vi "Front_Panel_Basic.vi"() -> ()   [LabVIEW 2015]
uses:
  Program Files (x86)/National Instruments/LabVIEW 2012/examples/Vision/2. Functions/Caliper/Control 1.ctl
panel:
  in  "Reset Sensor":bool
  in  "Set all":bool
  in  "Digital Offset Get":bool caption="Line Period Get"
  in  "Digital Offset Set":bool caption="Line Period Set"
  in  "Digital Offset":i16 min=-4096 max=4095 step=1
  in  "Digital Gain Get":bool caption="Line Period Get"
  in  "Digital Gain Set":bool caption="Line Period Set"
  in  "Digital Gain":i16 min=0 max=1791 step=1
  in  "Analog Gain Get":bool caption="Line Period Get"
  in  "Analog Gain Set":bool caption="Line Period Set"
  in  "Analog Gain":u16 max=2
  in  "Trigger Modes Get":bool caption="Line Period Get"
  in  "Trigger Modes Set":bool caption="Line Period Set"
  in  "Trigger Modes":u16 max=3
  in  "Exposure Time Get":bool caption="Line Period Get"
  in  "Exposure Time Set":bool caption="Line Period Set"
  in  "Exposure Time":u16 min=1
  in  "Line Period Get":bool
  in  "Line Period Set":bool
  in  "Line Period":T1=1 min=1 step=1
  out "Sensor width":string
  out "Firmware version":string
  out "User defined name":string
  out "Serial number":string
  out "Manufactuer info":string
  out "Device version":string
  out "Model Name":string
  out "Manufacturer name":string
  in  "Download Button":bool
  in  "EXIT":bool
  in  "Get All":bool
  out "IMAQ Session Out":refnum<k11>
  out "Error Output":errorcluster
  in  "error in (no error)":errorcluster
  # "Line period from 1 (0.01us) to 65535 (655,35 us) with\nstep size 1 (0.01us)."
  # "0: x1.0 gain\n1: x2.0 gain\n2: x4.0 gain"
  # "Exposure time from 1 (0.01us) to 65535 (655,35 us) with step size 1 (0.01us)."
  # "Digial gain from x1.0 (0) to x7.9961 (1791), with a \nstep size of 0x0.0039 (1)"
  # "0: Internal line trigger with programmable exposure time and line period\n1: Internal line trigger with max exporure time and programmable line period\n2: External line trigger with programmable exposure time\n3: External line trigger with maximum exposure time"
  # "Digial offset from -4096 to 4095 with a step size of 1\nin 12-bit mode.\nIn 11-bit mode, offset will be divided by 2.\nIn 10-bit mode, offset will be divided by 4."
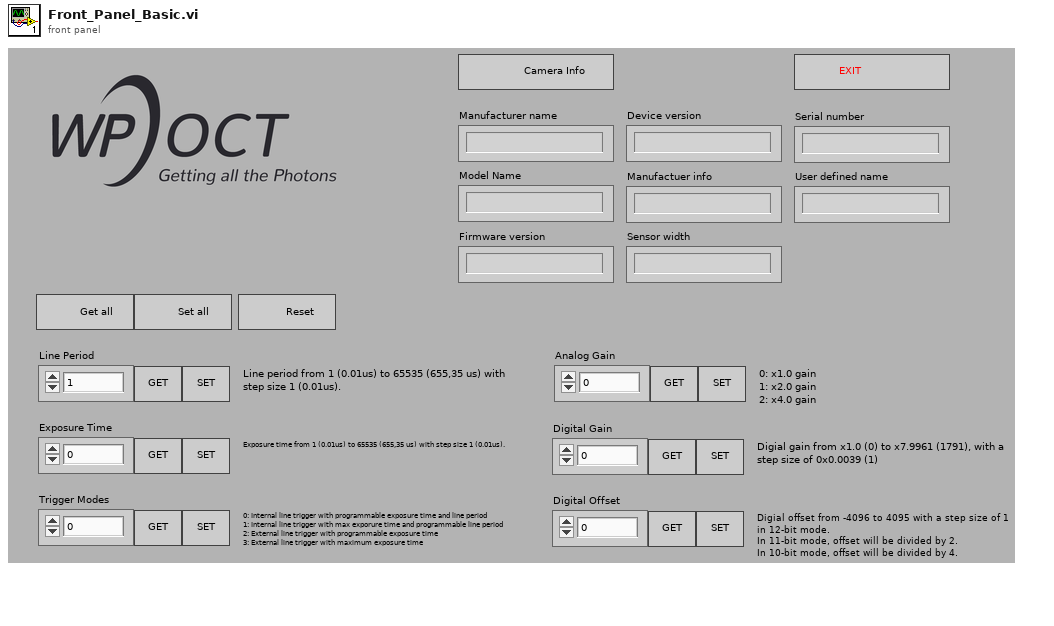
[diagram p1: front panel]
types:
  T1 = typedef "Control 1.ctl" = u16
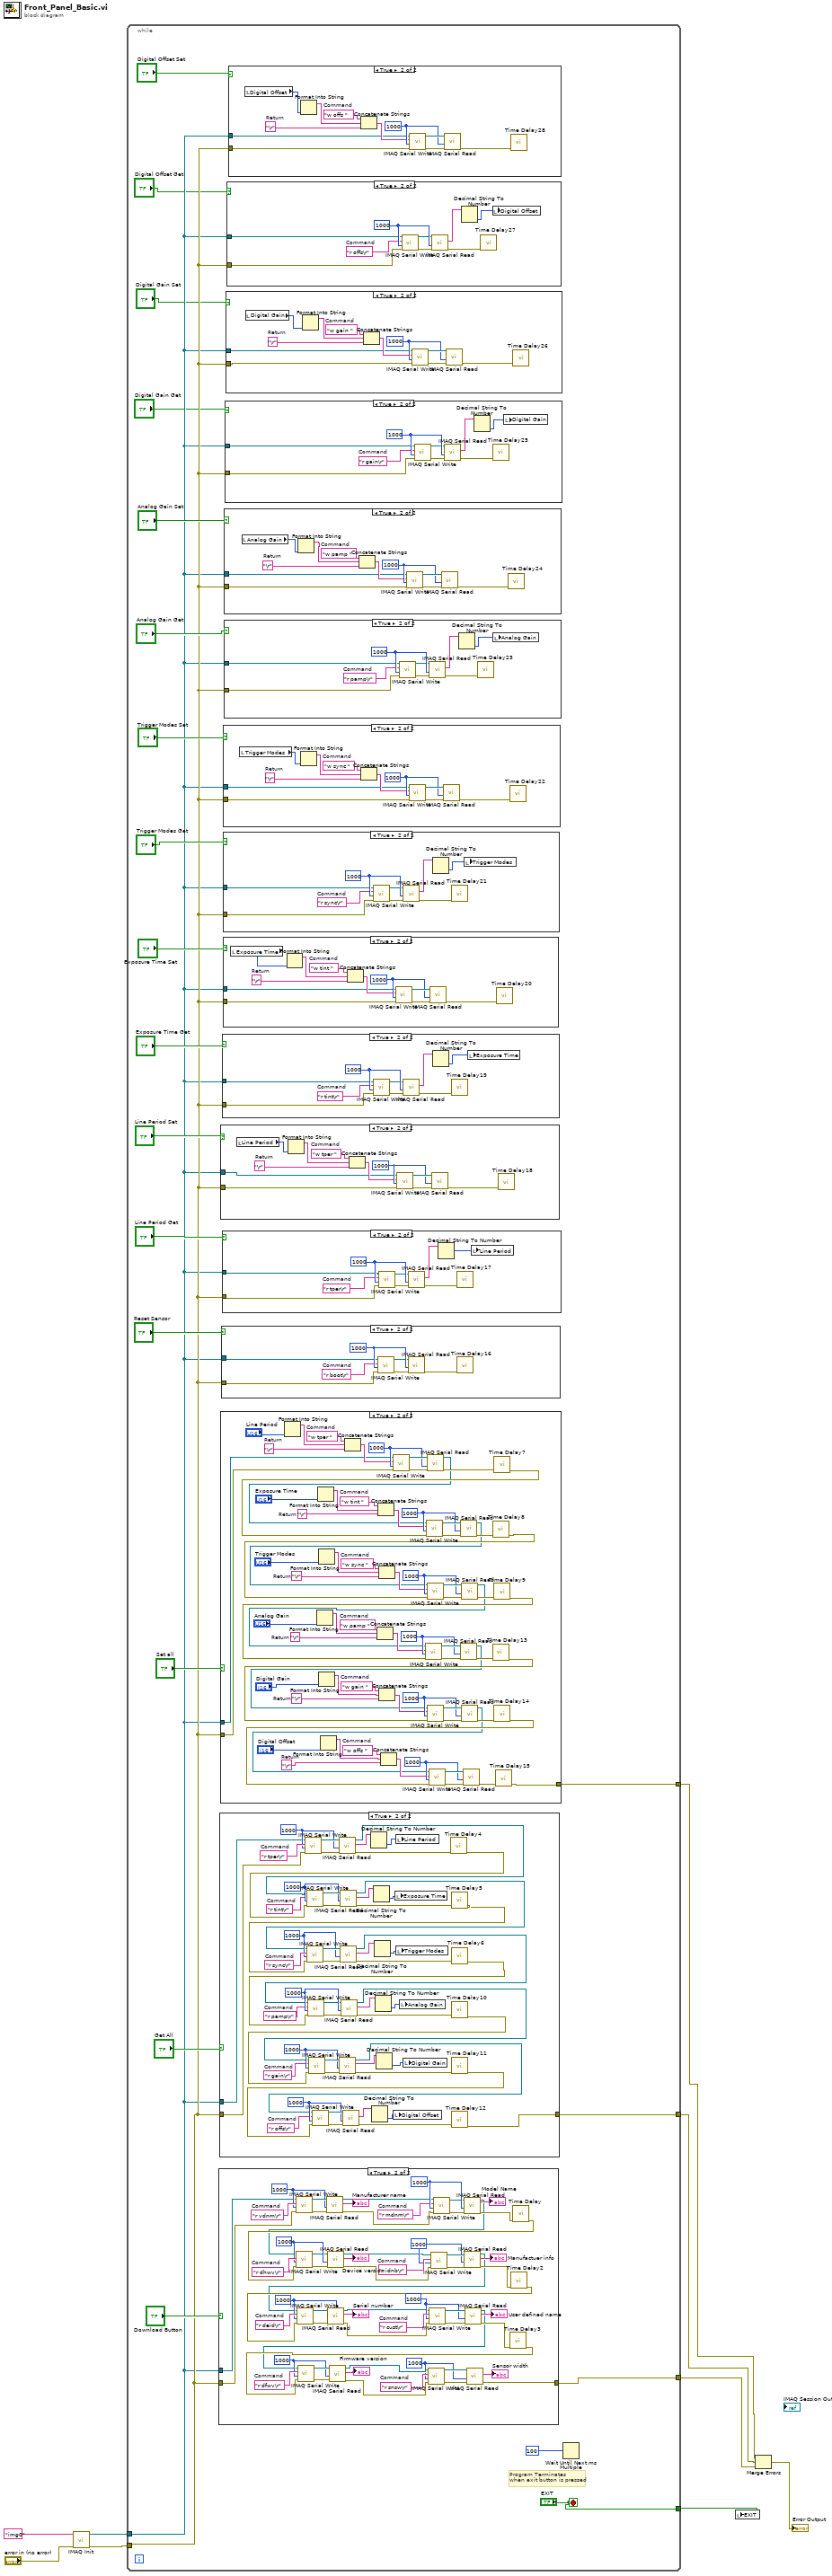
[diagram p0: block diagram]
diagram:
  n1 = call <vilib>:"IMAQ Init.vi"("error in (no error)"="error in (no error)", "Interface Name"="img0") -> ("error out"=w7:errorcluster, "IMAQ Session Out"=w8:refnum<k11>)  [unwired: 8 in]
  n2 = while {
    tunnel: w8 -> [w14]
    tunnel: w7 -> [w15]
    tunnel: ["EXIT"] -> w4
    tunnel: [w29] -> w3
    tunnel: [w26] -> w2
    tunnel: [w25] -> w1
    stop <- "EXIT" stop-if-true
    # "Program Terminates\nwhen exit button is pressed"
    n3 = case shown="True" "Download Button" {
      tunnel: w15 -> [w284 w307]
      tunnel: [w284 w285] -> w29
      tunnel: w14 -> [_ w306]
      frame False {
      }
      frame True {
        w310 = "r vdnm\r"  # Command
        w308 = 1000
        w316 = 1000
        w315 = "r mdnm\r"  # Command
        w320 = "r dhwv\r"  # Command
        w319 = 1000
        w322 = "r idnb\r"  # Command
        w321 = 1000
        w326 = 1000
        w327 = "r deid\r"  # Command
        w334 = "r cust\r"  # Command
        w331 = 1000
        w340 = "r dfwv\r"  # Command
        w336 = 1000
        w343 = "r snsw\r"  # Command
        w286 = 1000
        n4 = call <vilib>:"IMAQ Serial Write.vi"("error in (no error)"=w307, "Timeout"=w308, "String to write"=w310, "IMAQ Session In"=w306) -> ("error out"=w309:errorcluster, "IMAQ Session Out"=w311:refnum<k11>)  [unwired: 4 in]
        n5 = call <vilib>:"IMAQ Serial Read.vi"("error in (no error)"=w309, "Timeout"=w308, "IMAQ Session In"=w311) -> ("error out"=w303:errorcluster, "String Read"=→"Manufacturer name":string, "IMAQ Session Out"=w304:refnum<k11>)  [unwired: 3 in, 1 out]
        n6 = call <vilib>:"IMAQ Serial Write.vi"("error in (no error)"=w303, "Timeout"=w316, "String to write"=w315, "IMAQ Session In"=w304) -> ("error out"=w313:errorcluster, "IMAQ Session Out"=w312:refnum<k11>)  [unwired: 4 in]
        n7 = call <vilib>:"IMAQ Serial Read.vi"("error in (no error)"=w313, "Timeout"=w316, "IMAQ Session In"=w312) -> ("error out"=w302:errorcluster, "String Read"=→"Model Name":string, "IMAQ Session Out"=w300:refnum<k11>)  [unwired: 3 in, 1 out]
        n8 = call "Time Delay"("error in (no error)"=w302) -> ("error out"=w301:errorcluster)  [unwired: 10 in]
        n9 = call <vilib>:"IMAQ Serial Write.vi"("error in (no error)"=w301, "Timeout"=w319, "String to write"=w320, "IMAQ Session In"=w300) -> ("error out"=w318:errorcluster, "IMAQ Session Out"=w317:refnum<k11>)  [unwired: 4 in]
        n10 = call <vilib>:"IMAQ Serial Read.vi"("error in (no error)"=w318, "Timeout"=w319, "IMAQ Session In"=w317) -> ("error out"=w298:errorcluster, "String Read"=→"Device version":string, "IMAQ Session Out"=w297:refnum<k11>)  [unwired: 3 in, 1 out]
        n11 = call <vilib>:"IMAQ Serial Write.vi"("error in (no error)"=w298, "Timeout"=w321, "String to write"=w322, "IMAQ Session In"=w297) -> ("error out"=w323:errorcluster, "IMAQ Session Out"=w325:refnum<k11>)  [unwired: 4 in]
        n12 = call <vilib>:"IMAQ Serial Read.vi"("error in (no error)"=w323, "Timeout"=w321, "IMAQ Session In"=w325) -> ("error out"=w296:errorcluster, "String Read"=→"Manufactuer info":string, "IMAQ Session Out"=w294:refnum<k11>)  [unwired: 3 in, 1 out]
        n13 = call "Time Delay2"("error in (no error)"=w296) -> ("error out"=w295:errorcluster)  [unwired: 10 in]
        n14 = call <vilib>:"IMAQ Serial Write.vi"("error in (no error)"=w295, "Timeout"=w326, "String to write"=w327, "IMAQ Session In"=w294) -> ("error out"=w328:errorcluster, "IMAQ Session Out"=w329:refnum<k11>)  [unwired: 4 in]
        n15 = call <vilib>:"IMAQ Serial Read.vi"("error in (no error)"=w328, "Timeout"=w326, "IMAQ Session In"=w329) -> ("error out"=w289:errorcluster, "String Read"=→"Serial number":string, "IMAQ Session Out"=w293:refnum<k11>)  [unwired: 3 in, 1 out]
        n16 = call <vilib>:"IMAQ Serial Write.vi"("error in (no error)"=w289, "Timeout"=w331, "String to write"=w334, "IMAQ Session In"=w293) -> ("error out"=w332:errorcluster, "IMAQ Session Out"=w333:refnum<k11>)  [unwired: 4 in]
        n17 = call <vilib>:"IMAQ Serial Read.vi"("error in (no error)"=w332, "Timeout"=w331, "IMAQ Session In"=w333) -> ("error out"=w292:errorcluster, "String Read"=→"User defined name":string, "IMAQ Session Out"=w290:refnum<k11>)  [unwired: 3 in, 1 out]
        n18 = call "Time Delay3"("error in (no error)"=w292) -> ("error out"=w291:errorcluster)  [unwired: 10 in]
        n19 = call <vilib>:"IMAQ Serial Write.vi"("error in (no error)"=w291, "Timeout"=w336, "String to write"=w340, "IMAQ Session In"=w290) -> ("error out"=w337:errorcluster, "IMAQ Session Out"=w338:refnum<k11>)  [unwired: 4 in]
        n20 = call <vilib>:"IMAQ Serial Read.vi"("error in (no error)"=w337, "Timeout"=w336, "IMAQ Session In"=w338) -> ("error out"=w288:errorcluster, "String Read"=→"Firmware version":string, "IMAQ Session Out"=w287:refnum<k11>)  [unwired: 3 in, 1 out]
        n21 = call <vilib>:"IMAQ Serial Write.vi"("error in (no error)"=w288, "Timeout"=w286, "String to write"=w343, "IMAQ Session In"=w287) -> ("error out"=w342:errorcluster, "IMAQ Session Out"=w341:refnum<k11>)  [unwired: 4 in]
        n22 = call <vilib>:"IMAQ Serial Read.vi"("error in (no error)"=w342, "Timeout"=w286, "IMAQ Session In"=w341) -> ("error out"=w285:errorcluster, "String Read"=→"Sensor width":string)  [unwired: 3 in, 2 out]
      }
    }
    n23 = case shown="True" "Get All" {
      tunnel: w15 -> [w228 w279]
      tunnel: [w228 w234] -> w26
      tunnel: w14 -> [_ w278]
      frame False {
      }
      frame True {
        w236 = "r offs\r"  # Command
        w237 = 1000
        w260 = "r gain\r"  # Command
        w262 = 1000
        w265 = "r pamp\r"  # Command
        w266 = 1000
        w269 = "r sync\r"  # Command
        w250 = 1000
        w272 = "r tint\r"  # Command
        w274 = 1000
        w282 = "r tper\r"  # Command
        w280 = 1000
        n24 = call <vilib>:"IMAQ Serial Write.vi"("error in (no error)"=w279, "Timeout"=w280, "String to write"=w282, "IMAQ Session In"=w278) -> ("error out"=w281:errorcluster, "IMAQ Session Out"=w283:refnum<k11>)  [unwired: 4 in]
        n25 = call <vilib>:"IMAQ Serial Read.vi"("error in (no error)"=w281, "Timeout"=w280, "IMAQ Session In"=w283) -> ("error out"=w277:errorcluster, "String Read"=w241:string, "IMAQ Session Out"=w240:refnum<k11>)  [unwired: 3 in, 1 out]
        n26 = Decimal String To Number(string=w241) -> (number=w229:i32)  [unwired: 2 in, 1 out]
        n27 = local write "Line Period"(w229) -> ()
        n28 = call "Time Delay4"("error in (no error)"=w277) -> ("error out"=w242:errorcluster)  [unwired: 10 in]
        n29 = call <vilib>:"IMAQ Serial Write.vi"("error in (no error)"=w242, "Timeout"=w274, "String to write"=w272, "IMAQ Session In"=w240) -> ("error out"=w275:errorcluster, "IMAQ Session Out"=w276:refnum<k11>)  [unwired: 4 in]
        n30 = call <vilib>:"IMAQ Serial Read.vi"("error in (no error)"=w275, "Timeout"=w274, "IMAQ Session In"=w276) -> ("error out"=w273:errorcluster, "String Read"=w245:string, "IMAQ Session Out"=w243:refnum<k11>)  [unwired: 3 in, 1 out]
        n31 = Decimal String To Number(string=w245) -> (number=w244:i32)  [unwired: 2 in, 1 out]
        n32 = local write "Exposure Time"(w244) -> ()
        n33 = call "Time Delay5"("error in (no error)"=w273) -> ("error out"=w249:errorcluster)  [unwired: 10 in]
        n34 = call <vilib>:"IMAQ Serial Write.vi"("error in (no error)"=w249, "Timeout"=w250, "String to write"=w269, "IMAQ Session In"=w243) -> ("error out"=w270:errorcluster, "IMAQ Session Out"=w271:refnum<k11>)  [unwired: 4 in]
        n35 = call <vilib>:"IMAQ Serial Read.vi"("error in (no error)"=w270, "Timeout"=w250, "IMAQ Session In"=w271) -> ("error out"=w248:errorcluster, "String Read"=w247:string, "IMAQ Session Out"=w246:refnum<k11>)  [unwired: 3 in, 1 out]
        n36 = Decimal String To Number(string=w247) -> (number=w268:i32)  [unwired: 2 in, 1 out]
        n37 = local write "Trigger Modes"(w268) -> ()
        n38 = call "Time Delay6"("error in (no error)"=w248) -> ("error out"=w251:errorcluster)  [unwired: 10 in]
        n39 = call <vilib>:"IMAQ Serial Write.vi"("error in (no error)"=w251, "Timeout"=w266, "String to write"=w265, "IMAQ Session In"=w246) -> ("error out"=w267:errorcluster, "IMAQ Session Out"=w257:refnum<k11>)  [unwired: 4 in]
        n40 = call <vilib>:"IMAQ Serial Read.vi"("error in (no error)"=w267, "Timeout"=w266, "IMAQ Session In"=w257) -> ("error out"=w253:errorcluster, "String Read"=w255:string, "IMAQ Session Out"=w254:refnum<k11>)  [unwired: 3 in, 1 out]
        n41 = Decimal String To Number(string=w255) -> (number=w256:i32)  [unwired: 2 in, 1 out]
        n42 = local write "Analog Gain"(w256) -> ()
        n43 = call "Time Delay10"("error in (no error)"=w253) -> ("error out"=w252:errorcluster)  [unwired: 10 in]
        n44 = call <vilib>:"IMAQ Serial Write.vi"("error in (no error)"=w252, "Timeout"=w262, "String to write"=w260, "IMAQ Session In"=w254) -> ("error out"=w263:errorcluster, "IMAQ Session Out"=w264:refnum<k11>)  [unwired: 4 in]
        n45 = call <vilib>:"IMAQ Serial Read.vi"("error in (no error)"=w263, "Timeout"=w262, "IMAQ Session In"=w264) -> ("error out"=w261:errorcluster, "String Read"=w259:string, "IMAQ Session Out"=w232:refnum<k11>)  [unwired: 3 in, 1 out]
        n46 = Decimal String To Number(string=w259) -> (number=w258:i32)  [unwired: 2 in, 1 out]
        n47 = local write "Digital Gain"(w258) -> ()
        n48 = call "Time Delay11"("error in (no error)"=w261) -> ("error out"=w233:errorcluster)  [unwired: 10 in]
        n49 = call <vilib>:"IMAQ Serial Write.vi"("error in (no error)"=w233, "Timeout"=w237, "String to write"=w236, "IMAQ Session In"=w232) -> ("error out"=w238:errorcluster, "IMAQ Session Out"=w239:refnum<k11>)  [unwired: 4 in]
        n50 = call <vilib>:"IMAQ Serial Read.vi"("error in (no error)"=w238, "Timeout"=w237, "IMAQ Session In"=w239) -> ("error out"=w235:errorcluster, "String Read"=w231:string)  [unwired: 3 in, 2 out]
        n51 = Decimal String To Number(string=w231) -> (number=w230:i32)  [unwired: 2 in, 1 out]
        n52 = local write "Digital Offset"(w230) -> ()
        n53 = call "Time Delay12"("error in (no error)"=w235) -> ("error out"=w234:errorcluster)  [unwired: 10 in]
      }
    }
    n54 = case shown="True" "Set all" {
      tunnel: w15 -> [w160 w219]
      tunnel: [w160 w161] -> w25
      tunnel: w14 -> [_ w220]
      frame False {
      }
      frame True {
        w163 = "\r"  # Return
        w169 = "w offs "  # Command
        w170 = 1000
        w175 = "\r"  # Return
        w180 = "w gain "  # Command
        w181 = 1000
        w188 = "\r"  # Return
        w191 = "w pamp "  # Command
        w192 = 1000
        w196 = "\r"  # Return
        w201 = "w sync "  # Command
        w203 = 1000
        w213 = "\r"  # Return
        w211 = "w tint "  # Command
        w214 = 1000
        w224 = "\r"  # Return
        w222 = "w tper "  # Command
        w225 = 1000
        n55 = Format Into String("Line Period") -> (resulting string=w223:string)  [unwired: 3 in, 1 out]
        n56 = Format Into String("Analog Gain") -> (resulting string=w185:string)  [unwired: 3 in, 1 out]
        n57 = Format Into String("Exposure Time") -> (resulting string=w212:string)  [unwired: 3 in, 1 out]
        n58 = Format Into String("Trigger Modes") -> (resulting string=w202:string)  [unwired: 3 in, 1 out]
        n59 = Format Into String("Digital Gain") -> (resulting string=w174:string)  [unwired: 3 in, 1 out]
        n60 = Format Into String("Digital Offset") -> (resulting string=w162:string)  [unwired: 3 in, 1 out]
        n61 = Concatenate Strings(w222, w223, w224) -> (w221:string)
        n62 = Concatenate Strings(w191, w185, w188) -> (w190:string)
        n63 = Concatenate Strings(w211, w212, w213) -> (w210:string)
        n64 = Concatenate Strings(w201, w202, w196) -> (w200:string)
        n65 = Concatenate Strings(w180, w174, w175) -> (w179:string)
        n66 = Concatenate Strings(w169, w162, w163) -> (w168:string)
        n67 = call <vilib>:"IMAQ Serial Write.vi"("error in (no error)"=w219, "Timeout"=w225, "String to write"=w221, "IMAQ Session In"=w220) -> ("error out"=w226:errorcluster, "IMAQ Session Out"=w227:refnum<k11>)  [unwired: 4 in]
        n68 = call <vilib>:"IMAQ Serial Read.vi"("error in (no error)"=w226, "Timeout"=w225, "IMAQ Session In"=w227) -> ("error out"=w217:errorcluster, "IMAQ Session Out"=w206:refnum<k11>)  [unwired: 3 in, 2 out]
        n69 = call "Time Delay7"("error in (no error)"=w217) -> ("error out"=w207:errorcluster)  [unwired: 10 in]
        n70 = call <vilib>:"IMAQ Serial Write.vi"("error in (no error)"=w207, "Timeout"=w214, "String to write"=w210, "IMAQ Session In"=w206) -> ("error out"=w215:errorcluster, "IMAQ Session Out"=w216:refnum<k11>)  [unwired: 4 in]
        n71 = call <vilib>:"IMAQ Serial Read.vi"("error in (no error)"=w215, "Timeout"=w214, "IMAQ Session In"=w216) -> ("error out"=w209:errorcluster, "IMAQ Session Out"=w197:refnum<k11>)  [unwired: 3 in, 2 out]
        n72 = call "Time Delay8"("error in (no error)"=w209) -> ("error out"=w198:errorcluster)  [unwired: 10 in]
        n73 = call <vilib>:"IMAQ Serial Write.vi"("error in (no error)"=w198, "Timeout"=w203, "String to write"=w200, "IMAQ Session In"=w197) -> ("error out"=w204:errorcluster, "IMAQ Session Out"=w205:refnum<k11>)  [unwired: 4 in]
        n74 = call <vilib>:"IMAQ Serial Read.vi"("error in (no error)"=w204, "Timeout"=w203, "IMAQ Session In"=w205) -> ("error out"=w199:errorcluster, "IMAQ Session Out"=w186:refnum<k11>)  [unwired: 3 in, 2 out]
        n75 = call "Time Delay9"("error in (no error)"=w199) -> ("error out"=w187:errorcluster)  [unwired: 10 in]
        n76 = call <vilib>:"IMAQ Serial Write.vi"("error in (no error)"=w187, "Timeout"=w192, "String to write"=w190, "IMAQ Session In"=w186) -> ("error out"=w193:errorcluster, "IMAQ Session Out"=w194:refnum<k11>)  [unwired: 4 in]
        n77 = call <vilib>:"IMAQ Serial Read.vi"("error in (no error)"=w193, "Timeout"=w192, "IMAQ Session In"=w194) -> ("error out"=w189:errorcluster, "IMAQ Session Out"=w176:refnum<k11>)  [unwired: 3 in, 2 out]
        n78 = call "Time Delay13"("error in (no error)"=w189) -> ("error out"=w177:errorcluster)  [unwired: 10 in]
        n79 = call <vilib>:"IMAQ Serial Write.vi"("error in (no error)"=w177, "Timeout"=w181, "String to write"=w179, "IMAQ Session In"=w176) -> ("error out"=w182:errorcluster, "IMAQ Session Out"=w183:refnum<k11>)  [unwired: 4 in]
        n80 = call <vilib>:"IMAQ Serial Read.vi"("error in (no error)"=w182, "Timeout"=w181, "IMAQ Session In"=w183) -> ("error out"=w178:errorcluster, "IMAQ Session Out"=w165:refnum<k11>)  [unwired: 3 in, 2 out]
        n81 = call "Time Delay14"("error in (no error)"=w178) -> ("error out"=w166:errorcluster)  [unwired: 10 in]
        n82 = call <vilib>:"IMAQ Serial Write.vi"("error in (no error)"=w166, "Timeout"=w170, "String to write"=w168, "IMAQ Session In"=w165) -> ("error out"=w171:errorcluster, "IMAQ Session Out"=w172:refnum<k11>)  [unwired: 4 in]
        n83 = call <vilib>:"IMAQ Serial Read.vi"("error in (no error)"=w171, "Timeout"=w170, "IMAQ Session In"=w172) -> ("error out"=w167:errorcluster)  [unwired: 3 in, 3 out]
        n84 = call "Time Delay15"("error in (no error)"=w167) -> ("error out"=w161:errorcluster)  [unwired: 10 in]
      }
    }
    n85 = case shown="True" "Line Period Set" {
      tunnel: w15 -> [_ w136]
      tunnel: w14 -> [_ w135]
      frame False {
      }
      frame True {
        w134 = "\r"  # Return
        w139 = "w tper "  # Command
        w141 = 1000
        n86 = local read "Line Period"() -> (w133:T1)
        n87 = Format Into String(w133) -> (resulting string=w140:string)  [unwired: 3 in, 1 out]
        n88 = Concatenate Strings(w139, w140, w134) -> (w138:string)
        n89 = call <vilib>:"IMAQ Serial Write.vi"("error in (no error)"=w136, "Timeout"=w141, "String to write"=w138, "IMAQ Session In"=w135) -> ("error out"=w142:errorcluster, "IMAQ Session Out"=w143:refnum<k11>)  [unwired: 4 in]
        n90 = call <vilib>:"IMAQ Serial Read.vi"("error in (no error)"=w142, "Timeout"=w141, "IMAQ Session In"=w143) -> ("error out"=w137:errorcluster)  [unwired: 3 in, 3 out]
        n91 = call "Time Delay18"("error in (no error)"=w137) -> ()  [unwired: 10 in, 1 out]
      }
    }
    n92 = case shown="True" "Reset Sensor" {
      tunnel: w14 -> [_ w154]
      tunnel: w15 -> [_ w153]
      frame False {
      }
      frame True {
        w159 = 1000
        w158 = "r boot\r"  # Command
        n93 = call <vilib>:"IMAQ Serial Write.vi"("error in (no error)"=w153, "Timeout"=w159, "String to write"=w158, "IMAQ Session In"=w154) -> ("error out"=w157:errorcluster, "IMAQ Session Out"=w156:refnum<k11>)  [unwired: 4 in]
        n94 = call <vilib>:"IMAQ Serial Read.vi"("error in (no error)"=w157, "Timeout"=w159, "IMAQ Session In"=w156) -> ("error out"=w155:errorcluster)  [unwired: 3 in, 3 out]
        n95 = call "Time Delay16"("error in (no error)"=w155) -> ()  [unwired: 10 in, 1 out]
      }
    }
    n96 = case shown="True" "Exposure Time Get" {
      tunnel: w15 -> [_ w126]
      tunnel: w14 -> [_ w125]
      frame False {
      }
      frame True {
        w132 = 1000
        w124 = "r tint\r"  # Command
        n97 = call <vilib>:"IMAQ Serial Write.vi"("error in (no error)"=w126, "Timeout"=w132, "String to write"=w124, "IMAQ Session In"=w125) -> ("error out"=w131:errorcluster, "IMAQ Session Out"=w130:refnum<k11>)  [unwired: 4 in]
        n98 = call <vilib>:"IMAQ Serial Read.vi"("error in (no error)"=w131, "Timeout"=w132, "IMAQ Session In"=w130) -> ("error out"=w129:errorcluster, "String Read"=w128:string)  [unwired: 3 in, 2 out]
        n99 = Decimal String To Number(string=w128) -> (number=w127:i32)  [unwired: 2 in, 1 out]
        n100 = call "Time Delay19"("error in (no error)"=w129) -> ()  [unwired: 10 in, 1 out]
        n101 = local write "Exposure Time"(w127) -> ()
      }
    }
    n102 = case shown="True" "Line Period Get" {
      tunnel: w14 -> [_ w147]
      tunnel: w15 -> [_ w146]
      frame False {
      }
      frame True {
        w152 = 1000
        w151 = "r tper\r"  # Command
        n103 = call <vilib>:"IMAQ Serial Write.vi"("error in (no error)"=w146, "Timeout"=w152, "String to write"=w151, "IMAQ Session In"=w147) -> ("error out"=w150:errorcluster, "IMAQ Session Out"=w149:refnum<k11>)  [unwired: 4 in]
        n104 = call <vilib>:"IMAQ Serial Read.vi"("error in (no error)"=w150, "Timeout"=w152, "IMAQ Session In"=w149) -> ("error out"=w148:errorcluster, "String Read"=w145:string)  [unwired: 3 in, 2 out]
        n105 = Decimal String To Number(string=w145) -> (number=w144:i32)  [unwired: 2 in, 1 out]
        n106 = call "Time Delay17"("error in (no error)"=w148) -> ()  [unwired: 10 in, 1 out]
        n107 = local write "Line Period"(w144) -> ()
      }
    }
    n108 = case shown="True" "Trigger Modes Get" {
      tunnel: w15 -> [_ w106]
      tunnel: w14 -> [_ w105]
      frame False {
      }
      frame True {
        w112 = 1000
        w111 = "r sync\r"  # Command
        n109 = call <vilib>:"IMAQ Serial Write.vi"("error in (no error)"=w106, "Timeout"=w112, "String to write"=w111, "IMAQ Session In"=w105) -> ("error out"=w110:errorcluster, "IMAQ Session Out"=w109:refnum<k11>)  [unwired: 4 in]
        n110 = call <vilib>:"IMAQ Serial Read.vi"("error in (no error)"=w110, "Timeout"=w112, "IMAQ Session In"=w109) -> ("error out"=w108:errorcluster, "String Read"=w107:string)  [unwired: 3 in, 2 out]
        n111 = Decimal String To Number(string=w107) -> (number=w104:i32)  [unwired: 2 in, 1 out]
        n112 = call "Time Delay21"("error in (no error)"=w108) -> ()  [unwired: 10 in, 1 out]
        n113 = local write "Trigger Modes"(w104) -> ()
      }
    }
    n114 = case shown="True" "Exposure Time Set" {
      tunnel: w15 -> [_ w116]
      tunnel: w14 -> [_ w115]
      frame False {
      }
      frame True {
        w114 = "\r"  # Return
        w119 = "w tint "  # Command
        w121 = 1000
        n115 = local read "Exposure Time"() -> (w113:u16)
        n116 = Format Into String(w113) -> (resulting string=w120:string)  [unwired: 3 in, 1 out]
        n117 = Concatenate Strings(w119, w120, w114) -> (w118:string)
        n118 = call <vilib>:"IMAQ Serial Write.vi"("error in (no error)"=w116, "Timeout"=w121, "String to write"=w118, "IMAQ Session In"=w115) -> ("error out"=w122:errorcluster, "IMAQ Session Out"=w123:refnum<k11>)  [unwired: 4 in]
        n119 = call <vilib>:"IMAQ Serial Read.vi"("error in (no error)"=w122, "Timeout"=w121, "IMAQ Session In"=w123) -> ("error out"=w117:errorcluster)  [unwired: 3 in, 3 out]
        n120 = call "Time Delay20"("error in (no error)"=w117) -> ()  [unwired: 10 in, 1 out]
      }
    }
    n121 = case shown="True" "Trigger Modes Set" {
      tunnel: w15 -> [_ w96]
      tunnel: w14 -> [_ w95]
      frame False {
      }
      frame True {
        w97 = "\r"  # Return
        w100 = "w sync "  # Command
        w101 = 1000
        n122 = local read "Trigger Modes"() -> (w94:u16)
        n123 = Format Into String(w94) -> (resulting string=w93:string)  [unwired: 3 in, 1 out]
        n124 = Concatenate Strings(w100, w93, w97) -> (w99:string)
        n125 = call <vilib>:"IMAQ Serial Write.vi"("error in (no error)"=w96, "Timeout"=w101, "String to write"=w99, "IMAQ Session In"=w95) -> ("error out"=w102:errorcluster, "IMAQ Session Out"=w103:refnum<k11>)  [unwired: 4 in]
        n126 = call <vilib>:"IMAQ Serial Read.vi"("error in (no error)"=w102, "Timeout"=w101, "IMAQ Session In"=w103) -> ("error out"=w98:errorcluster)  [unwired: 3 in, 3 out]
        n127 = call "Time Delay22"("error in (no error)"=w98) -> ()  [unwired: 10 in, 1 out]
      }
    }
    n128 = case shown="True" "Analog Gain Set" {
      tunnel: w15 -> [_ w76]
      tunnel: w14 -> [_ w75]
      frame False {
      }
      frame True {
        w77 = "\r"  # Return
        w80 = "w pamp "  # Command
        w81 = 1000
        n129 = local read "Analog Gain"() -> (w73:u16)
        n130 = Format Into String(w73) -> (resulting string=w74:string)  [unwired: 3 in, 1 out]
        n131 = Concatenate Strings(w80, w74, w77) -> (w79:string)
        n132 = call <vilib>:"IMAQ Serial Write.vi"("error in (no error)"=w76, "Timeout"=w81, "String to write"=w79, "IMAQ Session In"=w75) -> ("error out"=w82:errorcluster, "IMAQ Session Out"=w83:refnum<k11>)  [unwired: 4 in]
        n133 = call <vilib>:"IMAQ Serial Read.vi"("error in (no error)"=w82, "Timeout"=w81, "IMAQ Session In"=w83) -> ("error out"=w78:errorcluster)  [unwired: 3 in, 3 out]
        n134 = call "Time Delay24"("error in (no error)"=w78) -> ()  [unwired: 10 in, 1 out]
      }
    }
    n135 = case shown="True" "Analog Gain Get" {
      tunnel: w15 -> [_ w86]
      tunnel: w14 -> [_ w85]
      frame False {
      }
      frame True {
        w92 = 1000
        w91 = "r pamp\r"  # Command
        n136 = call <vilib>:"IMAQ Serial Write.vi"("error in (no error)"=w86, "Timeout"=w92, "String to write"=w91, "IMAQ Session In"=w85) -> ("error out"=w90:errorcluster, "IMAQ Session Out"=w89:refnum<k11>)  [unwired: 4 in]
        n137 = call <vilib>:"IMAQ Serial Read.vi"("error in (no error)"=w90, "Timeout"=w92, "IMAQ Session In"=w89) -> ("error out"=w88:errorcluster, "String Read"=w87:string)  [unwired: 3 in, 2 out]
        n138 = Decimal String To Number(string=w87) -> (number=w84:i32)  [unwired: 2 in, 1 out]
        n139 = call "Time Delay23"("error in (no error)"=w88) -> ()  [unwired: 10 in, 1 out]
        n140 = local write "Analog Gain"(w84) -> ()
      }
    }
    n141 = case shown="True" "Digital Gain Get" {
      tunnel: w15 -> [_ w65]
      tunnel: w14 -> [_ w64]
      frame False {
      }
      frame True {
        w72 = 1000
        w71 = "r gain\r"  # Command
        n142 = call <vilib>:"IMAQ Serial Write.vi"("error in (no error)"=w65, "Timeout"=w72, "String to write"=w71, "IMAQ Session In"=w64) -> ("error out"=w70:errorcluster, "IMAQ Session Out"=w69:refnum<k11>)  [unwired: 4 in]
        n143 = call <vilib>:"IMAQ Serial Read.vi"("error in (no error)"=w70, "Timeout"=w72, "IMAQ Session In"=w69) -> ("error out"=w68:errorcluster, "String Read"=w66:string)  [unwired: 3 in, 2 out]
        n144 = Decimal String To Number(string=w66) -> (number=w67:i32)  [unwired: 2 in, 1 out]
        n145 = call "Time Delay25"("error in (no error)"=w68) -> ()  [unwired: 10 in, 1 out]
        n146 = local write "Digital Gain"(w67) -> ()
      }
    }
    n147 = case shown="True" "Digital Gain Set" {
      tunnel: w15 -> [_ w56]
      tunnel: w14 -> [_ w55]
      frame False {
      }
      frame True {
        w57 = "\r"  # Return
        w60 = "w gain "  # Command
        w61 = 1000
        n148 = local read "Digital Gain"() -> (w54:i16)
        n149 = Format Into String(w54) -> (resulting string=w53:string)  [unwired: 3 in, 1 out]
        n150 = Concatenate Strings(w60, w53, w57) -> (w59:string)
        n151 = call <vilib>:"IMAQ Serial Write.vi"("error in (no error)"=w56, "Timeout"=w61, "String to write"=w59, "IMAQ Session In"=w55) -> ("error out"=w62:errorcluster, "IMAQ Session Out"=w63:refnum<k11>)  [unwired: 4 in]
        n152 = call <vilib>:"IMAQ Serial Read.vi"("error in (no error)"=w62, "Timeout"=w61, "IMAQ Session In"=w63) -> ("error out"=w58:errorcluster)  [unwired: 3 in, 3 out]
        n153 = call "Time Delay26"("error in (no error)"=w58) -> ()  [unwired: 10 in, 1 out]
      }
    }
    n154 = case shown="True" "Digital Offset Get" {
      tunnel: w15 -> [_ w45]
      tunnel: w14 -> [_ w44]
      frame False {
      }
      frame True {
        w52 = 1000
        w51 = "r offs\r"  # Command
        n155 = call <vilib>:"IMAQ Serial Write.vi"("error in (no error)"=w45, "Timeout"=w52, "String to write"=w51, "IMAQ Session In"=w44) -> ("error out"=w50:errorcluster, "IMAQ Session Out"=w49:refnum<k11>)  [unwired: 4 in]
        n156 = call <vilib>:"IMAQ Serial Read.vi"("error in (no error)"=w50, "Timeout"=w52, "IMAQ Session In"=w49) -> ("error out"=w48:errorcluster, "String Read"=w46:string)  [unwired: 3 in, 2 out]
        n157 = Decimal String To Number(string=w46) -> (number=w47:i32)  [unwired: 2 in, 1 out]
        n158 = call "Time Delay27"("error in (no error)"=w48) -> ()  [unwired: 10 in, 1 out]
        n159 = local write "Digital Offset"(w47) -> ()
      }
    }
    n160 = case shown="True" "Digital Offset Set" {
      tunnel: w15 -> [_ w36]
      tunnel: w14 -> [_ w35]
      frame False {
      }
      frame True {
        w37 = "\r"  # Return
        w40 = "w offs "  # Command
        w41 = 1000
        n161 = local read "Digital Offset"() -> (w33:i16)
        n162 = Format Into String(w33) -> (resulting string=w34:string)  [unwired: 3 in, 1 out]
        n163 = Concatenate Strings(w40, w34, w37) -> (w39:string)
        n164 = call <vilib>:"IMAQ Serial Write.vi"("error in (no error)"=w36, "Timeout"=w41, "String to write"=w39, "IMAQ Session In"=w35) -> ("error out"=w42:errorcluster, "IMAQ Session Out"=w43:refnum<k11>)  [unwired: 4 in]
        n165 = call <vilib>:"IMAQ Serial Read.vi"("error in (no error)"=w42, "Timeout"=w41, "IMAQ Session In"=w43) -> ("error out"=w38:errorcluster)  [unwired: 3 in, 3 out]
        n166 = call "Time Delay28"("error in (no error)"=w38) -> ()  [unwired: 10 in, 1 out]
      }
    }
    n167 = Wait Until Next ms Multiple(millisecond multiple=100) -> ()  [unwired: 1 out]
  }
  n168 = local write "EXIT"(w4) -> ()
  n169 = Merge Errors(w1, w2, w3) -> (→"Error Output":errorcluster)
